vi "Local Endpoint A.vi"() -> ()   [LabVIEW 2020]
uses:
  Communication/IP_Communication/typedefs/General Settings.ctl
  Communication/IP_Communication/typedefs/Endpoint Tag.ctl
  Communication VIs/Local/Local.lvlib
  Communication/IP_Communication/IP_Communication.lvclass
panel:
  in  "General Settings":T1={"Connection Name"="Local_Test", "Endpoint Tag"=enum."A"}
  in  "Stop VI":bool
  in  "Send Command":bool
  in  "Command ID":u16
  out "Command Rx":T3
  out "Timeout?":bool
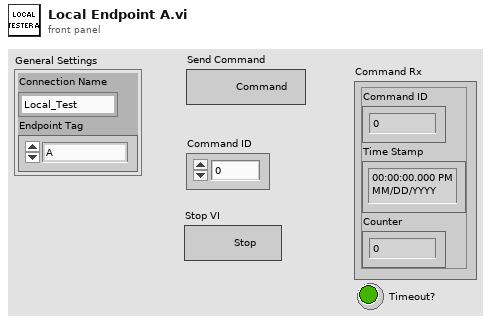
[diagram p1: front panel]
types:
  T1 = typedef "Communication Classes.lvlib/IP_Communication.lvclass/General Settings.ctl" = cluster{"Connection Name":string, "Endpoint Tag":T2}
  T2 = typedef "Communication Classes.lvlib/IP_Communication.lvclass/Endpoint Tag.ctl" = enum8{"A", "B"}
  T3 = cluster{"Command ID":u16, "Time Stamp":timestamp, "Counter":u16}
  T4 = cluster{"Command Out":cluster{"Command ID":u16, "Time Stamp":timestamp, "Counter":u16}, " Timeout?":bool}
  T5 = typedef "Communication VIs.lvlib/Local.lvlib/Local Queues.ctl" = cluster{"Rx_Queue":refnum<queue>, "Tx_Queue":refnum<queue>}
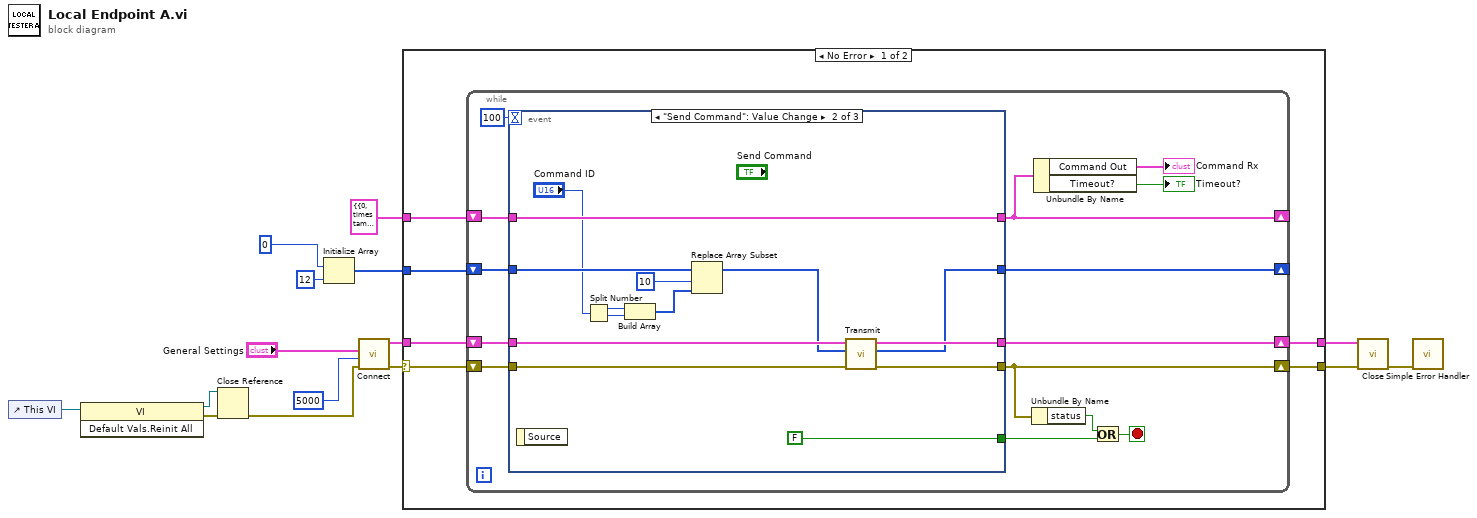
[diagram p0: block diagram]
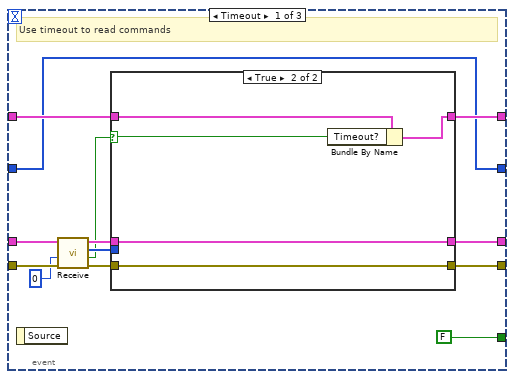
[diagram p2: hidden frame]
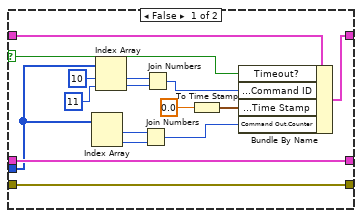
[diagram p3: hidden frame]
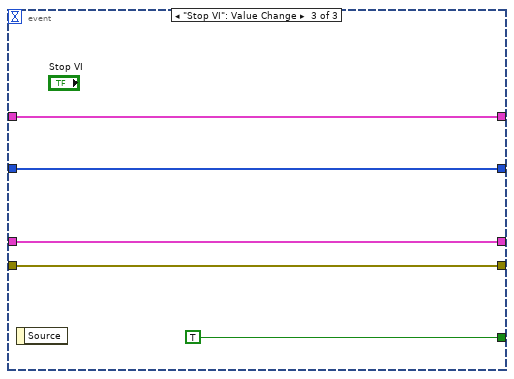
[diagram p4: hidden frame]
diagram:
  n1 = control-ref of="This VI"() -> (w12:refnum<vi>)
  n2 = invoke class="VI" method="Default Vals.Reinit All"(reference=w12) -> (reference out=w10:refnum<vi>, error out=w11:errorcluster)  [unwired: 2 in, 1 out]
  n3 = Close Reference(reference=w10, error in (no error)=w11) -> (error out=w5:errorcluster)
  n4 = Initialize Array(u8 0, 12 ("dimension size")) -> (w2:u8[])
  n5 = call "Connect.vi"("error in (no error)"=w5, "timeout in ms (10000)"=5000 ("Timeout"), "General Settings"="General Settings") -> ("error out"=w14:errorcluster, "Local Queues"=w13:T5)  [unwired: 7 in]
  n6 = case shown="No Error" w14 {
    selector: w14 -> [w21 w90]
    tunnel: [w18 w90] -> w8
    tunnel: [w17 w89] -> w1
    tunnel: w13 -> [w20 w89]
    tunnel: T4 {"Command Out"={"Command ID"=0, "Time Stamp"=timestamp(0 s since 1904-01-01), "Counter"=0}, " Timeout?"=FALSE} -> [w19 _]
    tunnel: w2 -> [w16 _]
    frame No Error {
      n7 = while {
        shift-right: [w30] -> _
        shift-left: w19 -> [w34]
        shift-right: [w31] -> w17
        shift-left: w20 -> [w33]
        shift-right: [w27] -> w18
        shift-left: w21 -> [w32]
        shift-right: [w22] -> _
        shift-left: w16 -> [w23]
        stop <- w26 stop-if-true
        n8 = event shown="[1] \"Send Command\": Value Change" {
          selector: _ -> [_ _ _]
          dyn-events: _ -> [_ _ _]
          timeout: 100 -> [_ _ _]
          tunnel: w34 -> [w40 w83 w88]
          tunnel: [w39 w83 w88] -> w30
          tunnel: w33 -> [w37 w80 w87]
          tunnel: w32 -> [w47 w72 w86]
          tunnel: [w45 w82 w86] -> w27
          tunnel: [w36 w71 w87] -> w31
          tunnel: [FALSE FALSE TRUE] -> w24
          tunnel: w23 -> [w38 w75 w84]
          tunnel: [w38 w70 w84] -> w22
          event Timeout {
            # "Use timeout to read commands"
            n9 = event-data() -> ()  [unwired: 1 in, 1 out]
            n10 = call "Receive.vi"("error in (no error)"=w47, "timeout in ms (0)"=0 ("timeout in ms (-1)"), "Local Queues in"=w37) -> ("error out"=w48:errorcluster, "Timeout?"=w41:bool, "Packet Received"=w43:u8[], "Local Queues out"=w46:T5)  [unwired: 5 in]
            n11 = case shown="True" w41 {
              selector: w41 -> [w62 w66]
              tunnel: w48 -> [w59 w68]
              tunnel: w46 -> [w61 w69]
              tunnel: [w59 w68] -> w45
              tunnel: [w61 w69] -> w36
              tunnel: w43 -> [w49 _]
              tunnel: w40 -> [w64 w67]
              tunnel: [w63 w65] -> w39
              frame False {
                n12 = Index Array(array=w49) -> (element #1=w57:u8, element #2=w56:u8)  [unwired: 2 in]
                n13 = Index Array(array=w49, index #1=10 ("index"), index #2=11 ("index")) -> (element #1=w53:u8, element #2=w54:u8)
                n14 = Join Numbers(hi=w57, lo=w56) -> ((hi.lo)=w55:u16)
                n15 = Join Numbers(hi=w53, lo=w54) -> ((hi.lo)=w50:u16)
                n16 = To Time Stamp(1:0.0 ("number")) -> (0:w60:timestamp)
                n17 = Bundle By Name(cluster=w64, "Timeout?"=w62, "Command Out.Command ID"=w50, "Command Out.Time Stamp"=w60, "Command Out.Counter"=w55) -> (w63:T4)
              }
              frame True {
                n18 = Bundle By Name(cluster=w67, "Timeout?"=w66) -> (w65:T4)
              }
            }
          }
          event "Send Command": Value Change {
            n19 = event-data() -> ()  [unwired: 1 in, 1 out]
            n20 = Split Number(x="Command ID") -> (hi(x)=w77:u8, lo(x)=w78:u8)
            n21 = Build Array(w77, w78) -> (w79:u8[])
            n22 = Replace Array Subset "Replace Array Subset"(array=w75, new element=w79, index=10) -> (w73:u8[])
            n23 = call "Transmit.vi"("error in (no error)"=w72, "Packet Data"=w73, "Local Queues in"=w80) -> ("error out"=w82:errorcluster, "Packet Data Sent"=w70:u8[], "Local Queues out"=w71:T5)  [unwired: 5 in, 1 out]
          }
          event "Stop VI": Value Change {
            n24 = event-data() -> ()  [unwired: 1 in, 1 out]
          }
        }
        n25 = Unbundle By Name(w27) -> ("status"=w25:bool)
        n26 = Unbundle By Name(w30) -> ("Command Out"=→"Command Rx":T3, "Timeout?"=→"Timeout?":bool)
        n27 = Or(x=w25, y=w24) -> (x .or. y?=w26:bool)
      }
    }
    frame Error {
    }
  }
  n28 = call "Close.vi"("error in (no error)"=w8, "Local Queues"=w1) -> ("error out"=w15:errorcluster)  [unwired: 9 in]
  n29 = call <vilib>:"Simple Error Handler.vi"("error in (no error)"=w15) -> ()  [unwired: 4 in, 5 out]
